vi "ROS_Master_lookupNodeReply.vi"(2 "node":string, 3 "ROS_Master in":T1) -> (0 "XML":string)   [LabVIEW 2012]
doc: "Returns XML from registering a node with the master"
uses:
  <userlib>/ROSforLV/ROS/Code/ROS_Master/ROS_Master.ctl
  <userlib>/ROSforLV/ROS/Code/ROS_Master/ROS_Topic.ctl
  <userlib>/ROSforLV/ROS/Code/ROS_Master/ROS_Node.ctl
  <userlib>/ROSforLV/ROS/Code/ROS_Master/ROS_Service.ctl
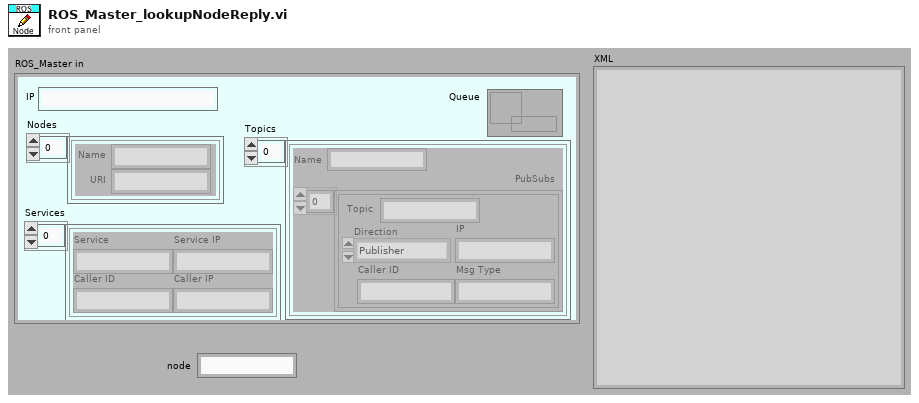
[diagram p1: front panel]
types:
  T1 = typedef "ROS_Master.ctl" = cluster{"IP":string, "Topics":cluster{"Name":string, "PubSubs":T2[]}[], "Nodes":T3[], "Services":T4[], "Queue":refnum<queue>}
  T2 = typedef "ROS_Topic.ctl" = cluster{"Caller ID":string, "IP":string, "Msg Type":string, "Direction":enum16{"Publisher", "Subscriber"}, "Topic":string}
  T3 = typedef "ROS_Node.ctl" = cluster{"Name":string, "URI":string}
  T4 = typedef "ROS_Service.ctl" = cluster{"Service":string, "Service IP":string, "Caller IP":string, "Caller ID":string}
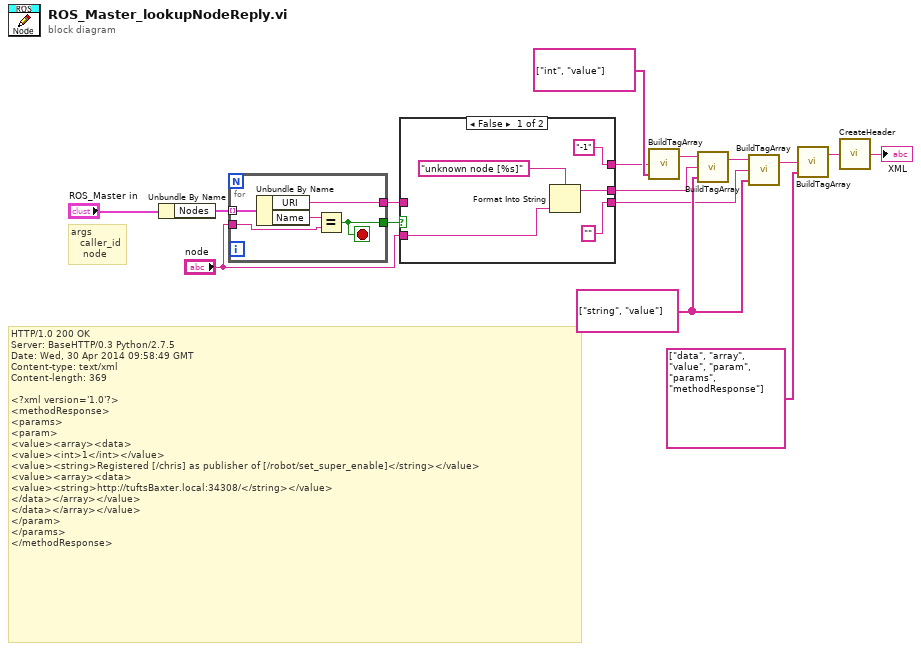
[diagram p0: block diagram]
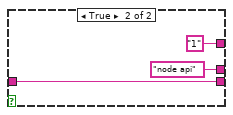
[diagram p2: hidden frame]
diagram:
  w7 = string[] ["string", "value"] ("tags")
  # "args\n   caller_id\n    node"
  # "HTTP/1.0 200 OK\nServer: BaseHTTP/0.3 Python/2.7.5\nDate: Wed, 30 Apr 2014 09:58:49 GMT\nContent-type: text/xml\nContent-length: 369\n\n<?xml version='1.0'?>\n<methodResponse>\n<params>\n<param>\n<value><array><data>\n<value><int>1</int></value>\n<value><string>Registered [/chris] as publisher of [/robot/set_super_enable]</string></value>\n<value><array><data>\n<value><string>http://tuftsBaxter.local:34308/</string></value>\n</data></array></value>\n</data></array></value>\n</param>\n</params>\n</methodResponse>"
  n1 = Unbundle By Name("ROS_Master in") -> ("Nodes"=w11:T3[])
  n2 = for {
    tunnel: w11 -> [w21] mode=indexing
    tunnel: "node" -> [w19]
    tunnel: [w18] -> w10
    tunnel: [w17] -> w9
    stop <- w18 stop-if-true
    n3 = Unbundle By Name(w21) -> ("URI"=w17:string, "Name"=w20:string)
    n4 = Equal?(x=w20, y=w19) -> (x = y?=w18:bool)
  }
  n5 = case shown="False" w10 {
    tunnel: w9 -> [_ w28]
    tunnel: "node" -> [w24 _]
    tunnel: ["-1" ("value") "1" ("value")] -> w5
    tunnel: ["" ("URI") w28] -> w4
    tunnel: [w23 "node api" ("value")] -> w3
    frame False {
      n6 = Format Into String(format string="unknown node [%s]", w24) -> (resulting string=w23:string)  [unwired: 2 in, 1 out]
    }
    frame True {
    }
  }
  n7 = call <userlib>:"BuildTagArray.vi"("tags"=string[] ["int", "value"], "value"=w5) -> ("string out"=w15:string)  [unwired: 2 in]
  n8 = call <userlib>:"BuildTagArray.vi"("tags"=w7, "value"=w3, "string in"=w15) -> ("string out"=w6:string)  [unwired: 1 in]
  n9 = call <userlib>:"BuildTagArray.vi"("tags"=w7, "value"=w4, "string in"=w6) -> ("string out"=w2:string)  [unwired: 1 in]
  n10 = call <userlib>:"BuildTagArray.vi"("tags"=string[] ["data", "array", "value", "param", "params", "methodResponse"], "value"=w2) -> ("string out"=w13:string)  [unwired: 2 in]
  n11 = call <userlib>:"CreateHeader.vi"("Content"=w13) -> ("XML"=→"XML":string)
